vi "Get Async Status.vi"(8 "error in (no error)":errorcluster, 10 "timeout in ms (0)":i32, 11 "queue in":refnum<queue>) -> (0 "error out":errorcluster, 2 "State":T1, 3 "queue out":refnum<queue>)   [LabVIEW 2011, in "Switch-DMM Custom Device.lvlib"]
uses:
  Switch-DMM Custom Device.lvlib
  Controls/Async Status.ctl
  Controls/Async State.ctl
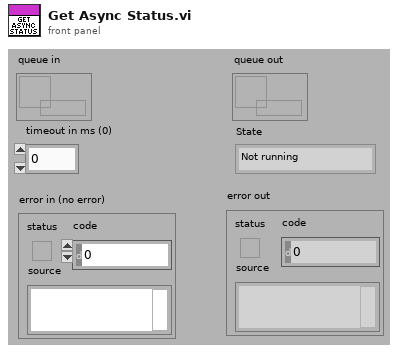
[diagram p1: front panel]
types:
  T1 = typedef "Switch-DMM Custom Device.lvlib/Async State.ctl" = enum16{"Not running", "Initializing", "Waiting on start cmd", "Running", "Stopped"}
  T2 = typedef "Switch-DMM Custom Device.lvlib/Async Status.ctl" = cluster{"State":T1, "error":errorcluster}
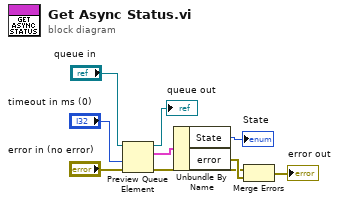
[diagram p0: block diagram]
diagram:
  n1 = Preview Queue Element(queue="queue in", timeout in ms (-1)="timeout in ms (0)", error in (no error)="error in (no error)") -> (queue out=→"queue out":refnum<queue>, element=w4:T2, error out=w7:errorcluster)  [unwired: 1 out]
  n2 = Unbundle By Name(w4) -> ("State"=→"State":T1, "error"=w8:errorcluster)
  n3 = Merge Errors(w7, w8) -> (→"error out":errorcluster)
